vi "ORS_get_alazar_acquisition_DLL_path.vi"(8 "error in (no error)":errorcluster) -> (0 "error out":errorcluster, 4 "Alazar Acquisition DLL path":path)   [LabVIEW 2024]
uses:
  <vilib>/Utility/error.llb/DialogType.ctl
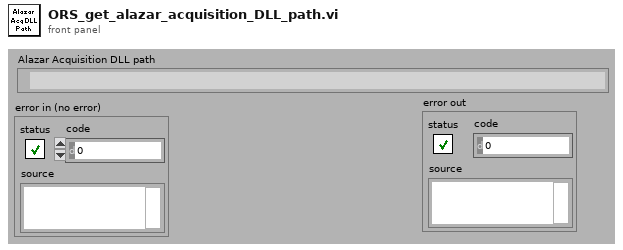
[diagram p1: front panel]
types:
  T1 = typedef "DialogType.ctl" = u16
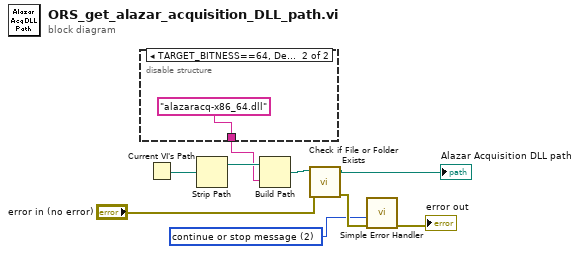
[diagram p0: block diagram]
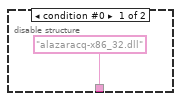
[diagram p2: hidden frame]
diagram:
  w2 = T1 2 items=["no dialog", "OK message", "continue or stop message", "OK message + warnings", "continue/stop + warnings"] ("type of dialog (OK msg:1)")
  n1 = disable-structure shown="TARGET_BITNESS==64, Default" {
    disable-tunnel: ["alazaracq-x86_32.dll" "alazaracq-x86_64.dll"] -> w7
    frame condition #0 {
    }
    frame condition #1 (active) {
    }
  }
  n2 = Current VI's Path() -> (path=w8:path)
  n3 = Strip Path(path=w8) -> (stripped path=w9:path)  [unwired: 1 out]
  n4 = Build Path(base path=w9, name or relative path=w7) -> (appended path=w6:path)
  n5 = call <vilib>:"Check if File or Folder Exists.vi"("error in (no error)"="error in (no error)", "path"=w6) -> ("error out"=w4:errorcluster, "dup path"=→"Alazar Acquisition DLL path":path)  [unwired: 7 in, 1 out]
  n6 = call <vilib>:"Simple Error Handler.vi"("type of dialog (OK msg:1)"=w2, "error in (no error)"=w4) -> ("error out"=→"error out":errorcluster)  [unwired: 3 in, 4 out]
